vi "Get Transaction by Row.vi"(8 "error in (no error)":errorcluster, 10 "Row":u32, 11 "Banking Statement in":refnum<class "Banking Statement.lvclass">) -> (0 "error out":errorcluster, 2 "Transaction.lvclass":refnum<class "Transaction.lvclass">, 3 "Banking Statement out":refnum<class "Banking Statement.lvclass">)   [LabVIEW 2018, in "Banking Statement.lvclass"]
uses:
  Banking Statement.lvclass
  Transaction/Transaction.lvclass
  Banking Statement.lvclass/Banking Statement.ctl
  Banking Record/Banking Transaction.lvclass
  C:/Users/jtipps/Documents/Filthy-Lucre-Budgetizer/source/support/classes/Transaction/Transaction.lvclass
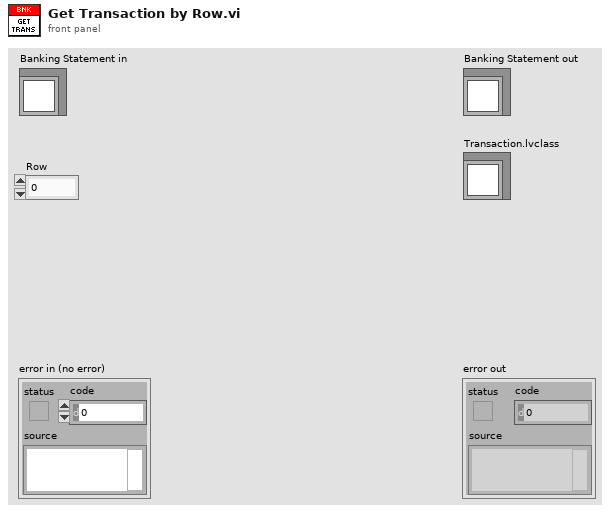
[diagram p1: front panel]
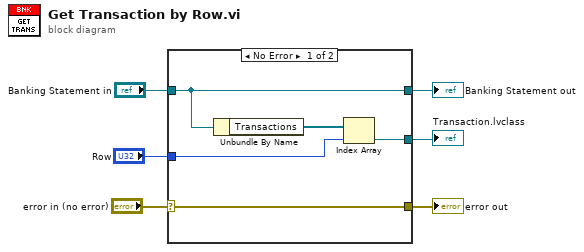
[diagram p0: block diagram]
diagram:
  n1 = case shown="No Error" "error in (no error)" {
    selector: "error in (no error)" -> [w8 w12]
    tunnel: "Banking Statement in" -> [w7 w13]
    tunnel: "Row" -> [w10 _]
    tunnel: [w9 _] -> w4
    tunnel: [w8 w12] -> w2
    tunnel: [w7 w13] -> w1
    frame No Error {
      n2 = Unbundle By Name(w7) -> ("Transactions"=w11:refnum<class "Banking Transaction.lvclass">[])
      n3 = Index Array(array=w11, index=w10) -> (element=w9:refnum<class "Banking Transaction.lvclass">)
    }
    frame Error {
    }
  }
  "error out" <- w2
  "Banking Statement out" <- w1
  "Transaction.lvclass" <- w4
